vi "Set Next Address.vi"(6 "physical":i32, 7 "length":i32, 8 "error in (no error)":errorcluster, 9 "highAdd":i32, 10 "lowAdd":i32, 11 "data":i32) -> (0 "error out":errorcluster, 2 "function return":u32, 3 "data out":i32)   [LabVIEW 2014, in "atmcd32d.lvlib"]
doc: "unsigned int WINAPI SetNextAddress(at_32 * data, long lowAdd, long highAdd, long length, long physical);"
uses:
  atmcd32d.lvlib
  atmcd32d.dll
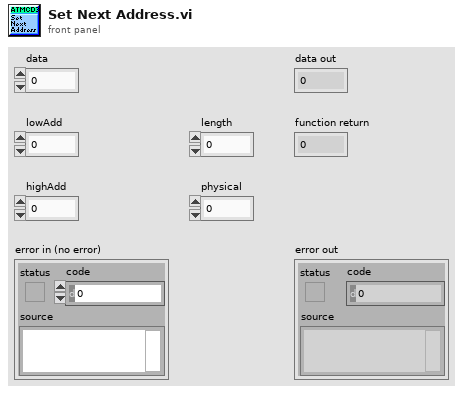
[diagram p1: front panel]
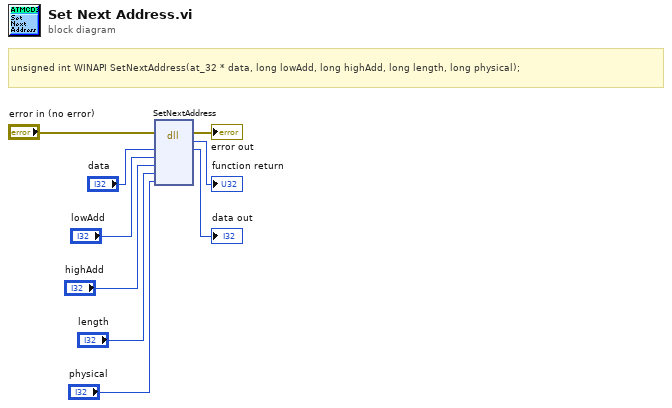
[diagram p0: block diagram]
diagram:
  # "unsigned int WINAPI SetNextAddress(at_32 * data, long lowAdd, long highAdd, long length, long physical);"
  n1 = dll-call lib="C:/Users/Bakir/Documents/Lambda2-Testing/lib/Andorlib/atmcd32d.*" fn="SetNextAddress"(error in="error in (no error)", "data"="data", "lowAdd"="lowAdd", "highAdd"="highAdd", "length"="length", "physical"="physical") -> (error out=→"error out":errorcluster, →"function return":u32, "data"=→"data out":i32)  [unwired: 6 in, 1 out]
